vi "Write Title.vi"(8 "error in (no error)":errorcluster, 10 "Title":refnum<vi>, 11 "Measurement in":refnum<class "Measurement.lvclass">) -> (0 "error out":errorcluster, 3 "Measurement out":refnum<class "Measurement.lvclass">)   [LabVIEW 2015, in "Measurement Actor.lvlib" / "Measurement.lvclass"]
uses:
  Measurement.lvclass
  Measurement.lvclass/Measurement.ctl
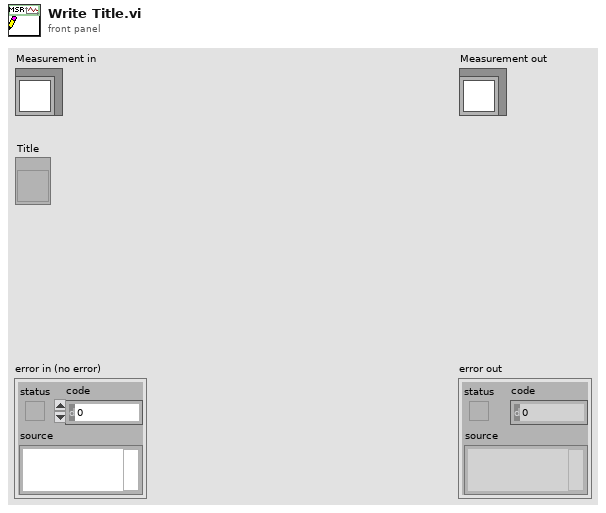
[diagram p1: front panel]
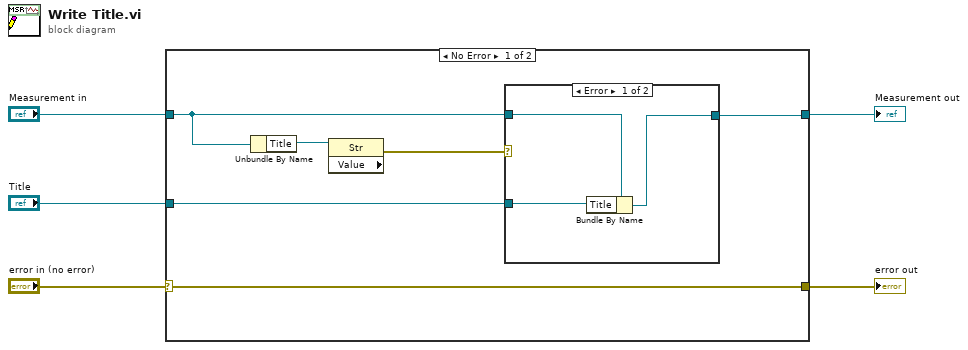
[diagram p0: block diagram]
diagram:
  n1 = case shown="No Error" "error in (no error)" {
    selector: "error in (no error)" -> [w11 w16]
    tunnel: [w11 w16] -> w4
    tunnel: [w6 w17] -> w2
    tunnel: "Measurement in" -> [w8 w17]
    tunnel: "Title" -> [w7 _]
    frame No Error {
      n2 = Unbundle By Name(w8) -> ("Title"=w9:refnum<vi>)
      n3 = property class="Str" props=["Value"](reference=w9) -> (error out=w10:errorcluster)  [unwired: 1 in, 2 out]
      n4 = case shown="Error" w10 {
        tunnel: [w14 w15] -> w6
        tunnel: w8 -> [w13 w15]
        tunnel: w7 -> [w12 _]
        frame Error {
          n5 = Bundle By Name(cluster=w13, "Title"=w12) -> (w14:refnum<class "Measurement.lvclass">)
        }
        frame No Error {
        }
      }
    }
    frame Error {
    }
  }
  "error out" <- w4
  "Measurement out" <- w2
